vi "measurementGlobal.vi"() -> ()   [LabVIEW 2013]
uses:
  Controls/saveDataOption.ctl
panel:
  in  "Tab Control":T1(tab)
  in  "Sampling Period (s)":dbl
  in  "Sampling Technique":string(combo)
  in  "Output No of samples":i32
  in  "Acquisition Card Kernel.vi":string(combo)
  in  "Iteration Num.":i32
  in  "Block Index":i32
  in  "Input No of Blocks":i32
  in  "Input No of samples":i32
  in  "Input Sampling rate (Hz)":dbl
  in  "Actual Measurement time (mins)":dbl
  in  "Average time (mins)":dbl
  in  "Data Acquision":T2(ring)
  in  "File Path":path
  in  "Save Data Option":T3
  out "error out":errorcluster
  in  "Task Name":string
  out "Chan + Span Limit":T4(array[cluster]) {"input terminal configuration" items=["Default"=-1, "RSE"=10083, "NRSE"=10078, "Differential"=10106, "Pseudodifferential"=12529]}
  in  "Analogue Data (volts)":dbl[][](array[numeric])
  out "taskReadInputs":refnum<k21>
  in  "sample mode":i32(ring)=10178 items=["Finite Samples"=10178, "Continuous Samples"=10123, "Hardware Timed Single Point"=12522]
  in  "NI Device Name":string
  in  "Pressure Scanner Clock Chans.":T5(array[cluster])
  in  "Pressure Scanner Freq. (Hz)":dbl
  out "Signal Processing Type":cluster{"Signal Pro. Type":string}[](array[cluster])
  # "Sampling by time does not work properly"
  # "Note: The Scanner Clock has to be the first two channels before of Chell Clock.vi"
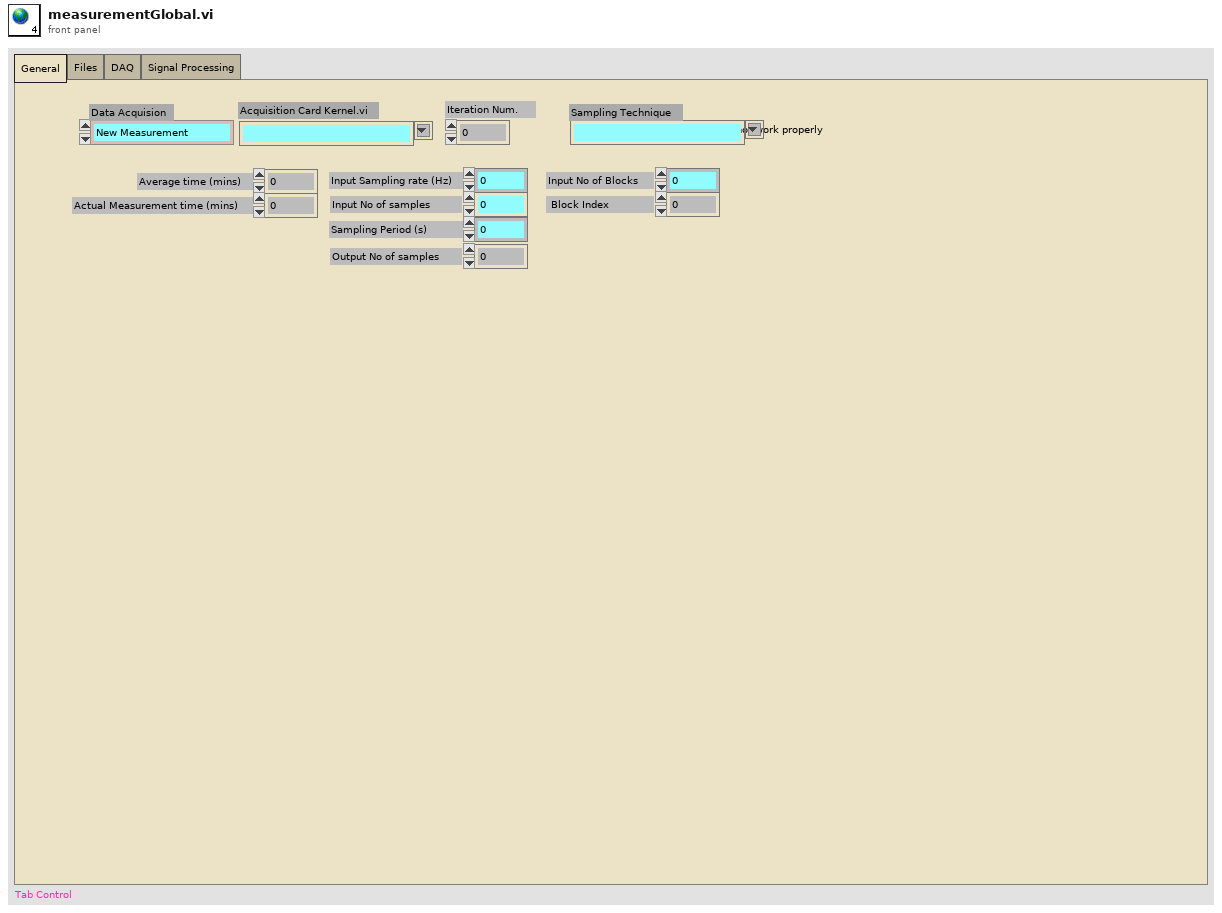
[diagram p1: front panel]
types:
  T1 = enum32{"General", "Files", "DAQ", "Signal Processing"}
  T2 = enum16{"New Measurement", "Post-process Raw Data"}
  T3 = typedef "saveDataOption.ctl" = enum16{"Save Data", "Do Not Save Data"}
  T4 = cluster{"Chan No.":i32, "Low Volt Limit (-10V)":dbl, "High Volt Limit (10V)":dbl, "input terminal configuration":i32}[]
  T5 = cluster{"Most Significant Bit":dbl, "Least Significant Bit":dbl}[]
diagram:
